vi "ThreeSessTwoPinThreeInstrTwoSiteReservation_CallNiDmmGetConnectionsNPinsMConnections_ReturnsThreeConnections.vi"(8 "error in":errorcluster) -> (0 "error out":errorcluster, 2 "result":string, 3 "pass":bool)   [LabVIEW 2020, in "MeasurementServerTests.lvlib"]
uses:
  MeasurementServerTests.lvlib
  Runtime/MeasurementLink Session Management/Session Reservation/Connection.ctl
  Runtime/MeasurementLink niDMM/Connection with Session.ctl
  f2d0f46c-20cf-4e81-b3a3-5c4fc317eda1.vi
  a536e905-e99b-4ce6-9f7b-add65bd26abc.vi
  03fc85e1-696b-4ece-a78b-f41470766ac0.vi
  b3e5c3be-b7a7-4b6e-86ee-709eea9cb752.vi
  Runtime/MeasurementLink niDMM/Get Connections - NPin NConn.vi
  Runtime/MeasurementLink Session Management/Session Reservation/Session Reservation.lvclass
  Runtime/MeasurementLink niDMM/MeasurementLink niDMM.lvlib
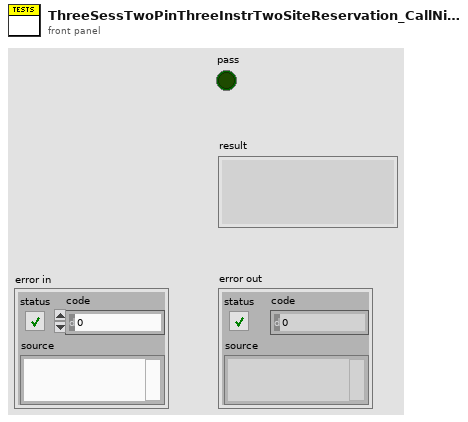
[diagram p1: front panel]
types:
  T1 = typedef "MeasurementLink niDMM.lvlib/Connection with Session.ctl" = cluster{"connection":T2, "session":refnum<k15>}
  T2 = typedef "MeasurementLink Session Management.lvlib/Session Reservation.lvclass/Connection.ctl" = cluster{"pin or relay name":string, "site":i32, "instrument type id":string, "channel":string}
  T3 = typedef "MeasurementLink Session Management.lvlib/Session Reservation.lvclass/Data.ctl" = cluster{"session and driver infos":T4[], "pin or relay names":string[]}
  T4 = typedef "MeasurementLink Session Management.lvlib/Session Reservation.lvclass/Session and Driver Info.ctl" = cluster{"session info":T5, "session":variant}
  T5 = typedef "MeasurementLink Session Management Client.lvlib/ni_measurementlink_sessionmanagement_v1_SessionInformation.ctl" = cluster{"session":T6, "resource_name":string, "channel_list":string, "instrument_type_id":string, "session_exists":bool, "channel_mappings":T7[]}
  T6 = typedef "MeasurementLink Session Management Client.lvlib/nidevice_grpc_Session.ctl" = cluster{"name":string}
  T7 = typedef "MeasurementLink Session Management Client.lvlib/ni_measurementlink_sessionmanagement_v1_ChannelMapping.ctl" = cluster{"pin_or_relay_name":string, "site":i32, "channel":string}
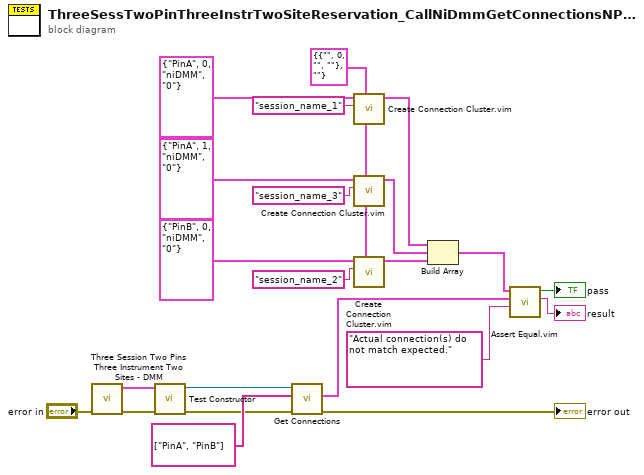
[diagram p0: block diagram]
diagram:
  w3 = T1 {"connection"={"pin or relay name"="", "site"=0, "instrument type id"="", "channel"=""}, "session"=""} ("connection with session")
  n1 = call "Three Session Two Pins Three Instrument Two Sites - DMM.vi"("error in"="error in") -> ("error out"=w5:errorcluster, "data out"=w6:T3)  [unwired: 9 in]
  n2 = call "Test Constructor.vi"("error in"=w5, "data"=w6) -> ("error out"=w9:errorcluster, "Session Reservation out"=w11:refnum<class "Session Reservation.lvclass">)  [unwired: 8 in]
  n3 = call-poly "Get Connections.vi"("error in"=w9, "pin or relay names"=string[] ["PinA", "PinB"], "session reservation in"=w11) -> ("error out"=→"error out":errorcluster, "connections"=w7:T1[])  [unwired: 6 in, 1 out]
  n4 = call "Create Connection Cluster.vim"("connection type"=w3, "session in"="session_name_1", "hardware independent connection in"=T2 {"pin or relay name"="PinA", "site"=0, "instrument type id"="niDMM", "channel"="0"} ("connection")) -> ("connection out"=w17:T1)  [unwired: 8 in]
  n5 = call "Create Connection Cluster.vim"("connection type"=w3, "session in"="session_name_3", "hardware independent connection in"=T2 {"pin or relay name"="PinA", "site"=1, "instrument type id"="niDMM", "channel"="0"} ("connection")) -> ("connection out"=w16:T1)  [unwired: 8 in]
  n6 = call "Create Connection Cluster.vim"("connection type"=w3, "session in"="session_name_2", "hardware independent connection in"=T2 {"pin or relay name"="PinB", "site"=0, "instrument type id"="niDMM", "channel"="0"} ("connection")) -> ("connection out"=w12:T1)  [unwired: 8 in]
  n7 = Build Array(w17, w16, w12) -> (w15:T1[])
  n8 = call "Assert Equal.vim"("failure message"="Actual connection(s) do not match expected.", "actual value"=w7, "expected value"=w15) -> ("message"=→"result":string, "equal?"=→"pass":bool)  [unwired: 7 in]
